vi "Configure Voltage Limit.vi"(8 "error in (no error)":errorcluster, 10 "Max Voltage Limit (61.000 V)":dbl=61.0 min=0.0 max=151.0 step=0.001 format="%.3f", 11 "VISA resource name":refnum<visa-resource-name>) -> (0 "error out":errorcluster, 3 "VISA resource name out":refnum<visa-resource-name>)   [LabVIEW 2023, in "BK Precision 9200 Series.lvlib"]
doc: "Configures the maximum output voltage limit."
uses:
  <instrlib>/BK Precision 9200 Series/BK Precision 9200 Series.lvlib
panel:
  # "V"
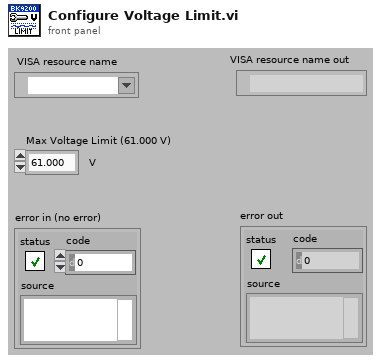
[diagram p1: front panel]
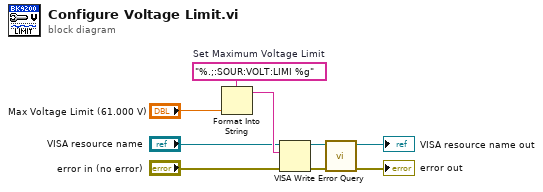
[diagram p0: block diagram]
diagram:
  w5 = "%.;:SOUR:VOLT:LIMI %g"  # Set Maximum Voltage Limit
  n1 = Format Into String(format string=w5, "Max Voltage Limit (61.000 V)") -> (resulting string=w3:string)  [unwired: 2 in, 1 out]
  n2 = VISA Write(VISA resource name="VISA resource name", write buffer=w3, error in (no error)="error in (no error)") -> (VISA resource name out=w6:refnum<visa-resource-name>, error out=w7:errorcluster)  [unwired: 1 out]
  n3 = call <instrlib>:"Error Query.vi"("error in (no error)"=w7, "VISA resource name"=w6) -> ("error out"=→"error out":errorcluster, "VISA resource name out"=→"VISA resource name out":refnum<visa-resource-name>)  [unwired: 6 in, 2 out]
